vi "Get VI Metrics.vi"(8 "error in (no error)":errorcluster, 10 "VI Path":path, 11 "Code Inspector in":refnum<class "Code Inspector.lvclass">) -> (0 "error out":errorcluster, 2 "VI Name":string, 3 "Code Inspector out":refnum<class "Code Inspector.lvclass">, 4 "Total Diagram Count":i32, 5 "Total Node Count":i32, 6 "Uncovered Diagram Count":i32, 7 "Uncovered Node Count":i32)   [LabVIEW 2017, in "Cobertura.lvlib" / "Code Inspector.lvclass"]
uses:
  Code Inspector.lvclass
  <vilib>/Utility/traverseref.llb/TRef TravTarget.ctl
  Code Inspector.lvclass/Code Inspector.ctl
  <vilib>/Utility/traverseref.llb/VI Scripting - Traverse.lvlib
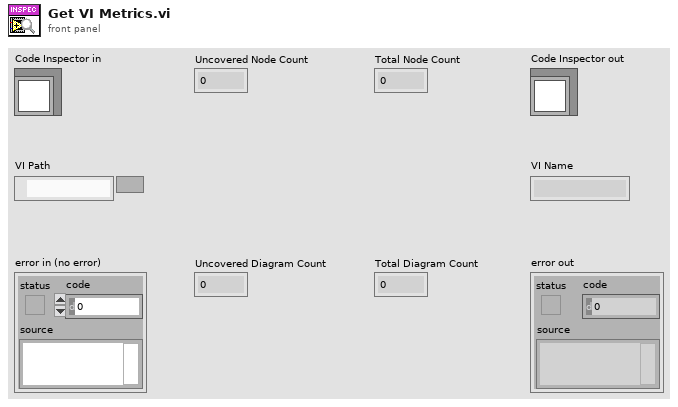
[diagram p1: front panel]
types:
  T1 = typedef "TRef TravTarget.ctl" = enum16{"FP", "BD", "Other"}
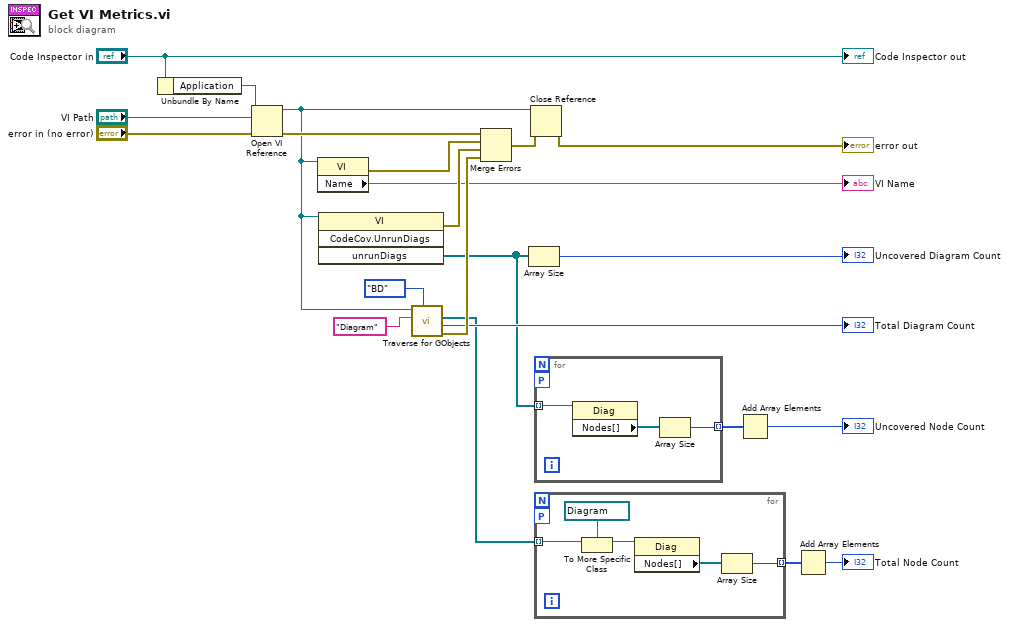
[diagram p0: block diagram]
diagram:
  n1 = Unbundle By Name("Code Inspector in") -> ("Application"=w18:refnum<vi>)
  n2 = Open VI Reference(application reference (local)=w18, vi path="VI Path", error in (no error)="error in (no error)") -> (vi reference=w7:refnum<vi>, error out=w15:errorcluster)  [unwired: 3 in]
  n3 = property class="VI"(reference=w7) -> (error out=w11:errorcluster, "Name"=→"VI Name":string)  [unwired: 1 in, 1 out]
  n4 = invoke class="VI" method="CodeCov.UnrunDiags"(reference=w7) -> (error out=w14:errorcluster, "unrunDiags"=w6:refnum<vi>[])  [unwired: 3 in, 2 out]
  n5 = call <vilib>:"Traverse for GObjects.vi"("Traverse Target"=TRef_TravTarget."BD", "Class Name"="Diagram", "VI Refnum"=w7) -> ("error out"=w13:errorcluster, "# of Refs"=→"Total Diagram Count":i32, "References"=w3:refnum<vi>[])  [unwired: 5 in, 1 out]
  n6 = Merge Errors(w15, w11, w14, w13) -> (w9:errorcluster)
  n7 = Array Size(array=w6) -> (size(s)=→"Uncovered Diagram Count":i32)
  n8 = Close Reference(reference=w7, error in (no error)=w9) -> (error out=→"error out":errorcluster)
  n9 = for {
    tunnel: w6 -> [w25] mode=indexing
    tunnel: [w23] -> w5 mode=indexing
    workers-P: _ -> [_]
    n10 = property class="Diag"(reference=w25) -> ("Nodes[]"=w24:refnum<vi>[])  [unwired: 1 in, 2 out]
    n11 = Array Size(array=w24) -> (size(s)=w23:i32)
  }
  n12 = for {
    tunnel: [w29] -> w4 mode=indexing
    workers-P: _ -> [_]
    tunnel: w3 -> [w26] mode=indexing
    n13 = To More Specific Class(target class=refnum<vi> refnum, reference=w26) -> (specific class reference=w27:refnum<vi>)  [unwired: 1 in, 1 out]
    n14 = property class="Diag"(reference=w27) -> ("Nodes[]"=w30:refnum<vi>[])  [unwired: 1 in, 2 out]
    n15 = Array Size(array=w30) -> (size(s)=w29:i32)
  }
  n16 = Add Array Elements(numeric array=w5) -> (sum=→"Uncovered Node Count":i32)
  n17 = Add Array Elements(numeric array=w4) -> (sum=→"Total Node Count":i32)
  "Code Inspector out" <- "Code Inspector in"
